vi "FileIO_Parse_ERD_XML.vi"(0 "ERD XML File":path, 11 "Error In":errorcluster) -> (4 "ERD Names":string[](array[string]), 6 "ERD Numbers":u16[](array[numeric]) format="%.0x", 8 "#ERDs Found":i32, 15 "Error Out":errorcluster)   [LabVIEW 2018]
uses:
  <vilib>/xml/Close Reference(Node).vi
  <resource>/objmgr/DOMUserDefRef.rc
  <vilib>/xml/NI_XML.lvlib
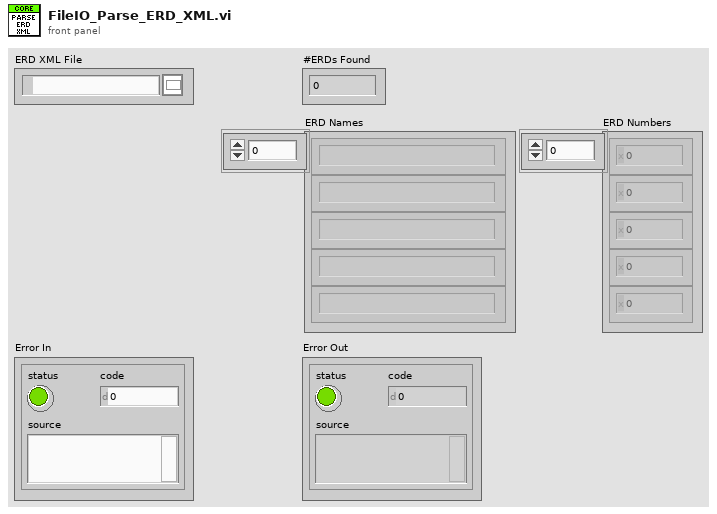
[diagram p1: front panel]
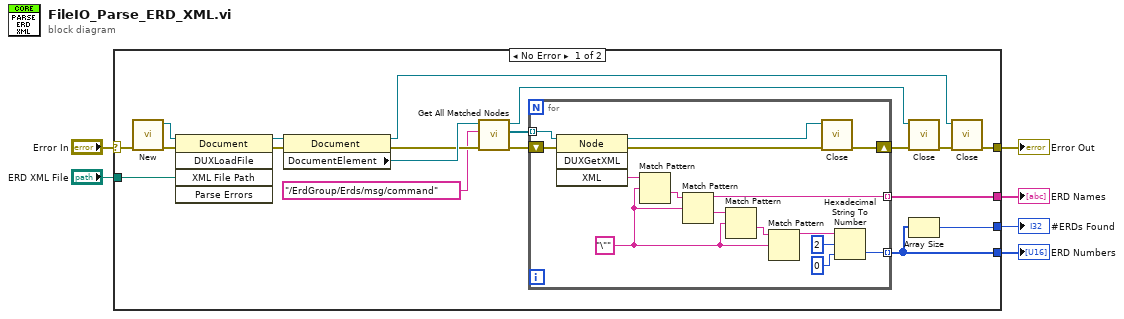
[diagram p0: block diagram]
diagram:
  n1 = case shown="No Error" "Error In" {
    selector: "Error In" -> [w11 w41]
    tunnel: "ERD XML File" -> [w24 _]
    tunnel: [w16 _] -> w5
    tunnel: [w10 _] -> w4
    tunnel: [w7 _] -> w3
    tunnel: [w8 w41] -> w2
    frame No Error {
      n2 = call <vilib>:"New.vi"("error in (no error)"=w11) -> ("error out"=w23:errorcluster, "DOM document out"=w25:refnum<k20>)  [unwired: 7 in]
      n3 = invoke class="Document" method="DUXLoadFile"(reference=w25, error in=w23, "XML File Path"=w24) -> (reference out=w18:refnum<k20>, error out=w17:errorcluster)  [unwired: 2 in, 3 out]
      n4 = property class="Document"(reference=w18, error in=w17) -> (reference out=w12:refnum<k20>, error out=w19:errorcluster, "DocumentElement"=w22:refnum<k20>)
      n5 = call <vilib>:"Get All Matched Nodes.vi"("error in (no error)"=w19, "XPath expression"="/ErdGroup/Erds/msg/command", "node in"=w22) -> ("error out"=w20:errorcluster, "node result array"=w21:refnum<k20>[], "node out"=w14:refnum<k20>)  [unwired: 6 in]
      n6 = for {
        tunnel: w21 -> [w39] mode=indexing
        shift-right: [w27] -> w9
        shift-left: w20 -> [w40]
        tunnel: [w35] -> w7 mode=indexing
        tunnel: [w32] -> w10 mode=indexing
        w26 = "\"" ("regular expression")
        n7 = invoke on="Invoke Node" class="Node" method="DUXGetXML"(reference=w39, error in=w40) -> (reference out=w37:refnum<k20>, error out=w38:errorcluster, "XML"=w34:string)  [unwired: 2 in, 1 out]
        n8 = Match Pattern(string=w34, regular expression=w26) -> (after substring=w33:string)  [unwired: 1 in, 3 out]
        n9 = Match Pattern(string=w33, regular expression=w26) -> (before substring=w32:string, after substring=w30:string)  [unwired: 1 in, 2 out]
        n10 = Match Pattern(string=w30, regular expression=w26) -> (after substring=w31:string)  [unwired: 1 in, 3 out]
        n11 = Match Pattern(string=w31, regular expression=w26) -> (before substring=w29:string)  [unwired: 1 in, 3 out]
        n12 = call-poly <vilib>:"Close.vi"("error in (no error)"=w38, "node"=w37) -> ("error out"=w27:errorcluster)  [unwired: 7 in]
        n13 = Hexadecimal String To Number(string=w29, offset=2, default (0uL)=u16 0 ("default (0 U32)")) -> (number=w35:u16)  [unwired: 1 out]
      }
      n14 = call-poly <vilib>:"Close.vi"("error in (no error)"=w9, "node"=w14) -> ("error out"=w13:errorcluster)  [unwired: 7 in]
      n15 = Array Size(array=w7) -> (size(s)=w16:i32)
      n16 = call-poly <vilib>:"Close.vi"("error in (no error)"=w13, "node"=w12) -> ("error out"=w8:errorcluster)  [unwired: 7 in]
    }
    frame Error {
    }
  }
  "#ERDs Found" <- w5
  "ERD Names" <- w4
  "ERD Numbers" <- w3
  "Error Out" <- w2
